vi "Box.vi"(4 "Position":cluster{"X":sgl, "Y":sgl, "Z":sgl}, 5 "Alpha":dbl=1.0, 7 "Color Box":u32(colorbox), 8 "error in (no error)":errorcluster, 9 "Size":T1, 10 "Name":string) -> (0 "error out":errorcluster, 3 "3D Object out":refnum<class "3D Object.lvclass">)   [LabVIEW 2015, in "3D Object.lvclass"]
uses:
  3D Object.lvclass
  <vilib>/picture/3D Picture Control/NI_3D Picture Control.lvlib
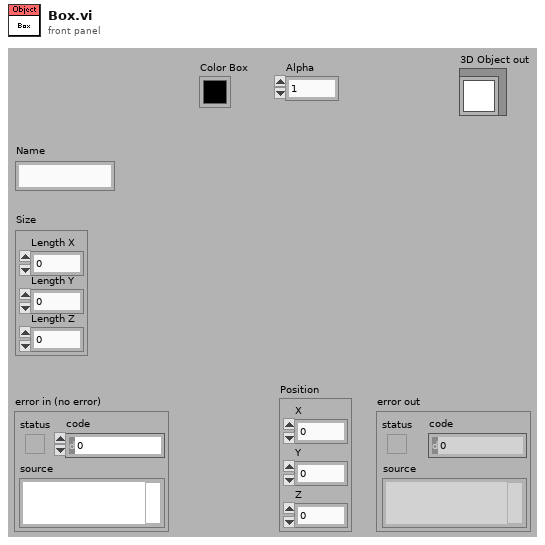
[diagram p1: front panel]
types:
  T1 = cluster{"Length X":sgl, "Length Y":sgl, "Length Z":sgl}
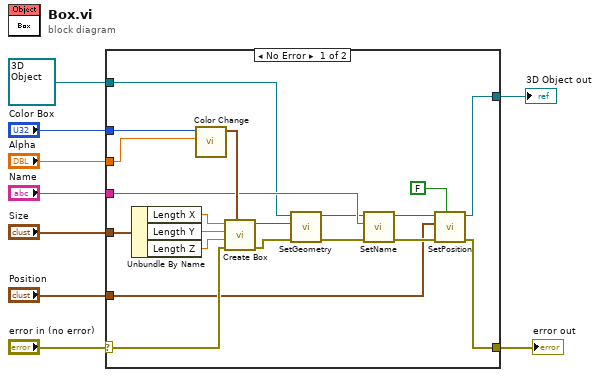
[diagram p0: block diagram]
diagram:
  n1 = case shown="No Error" "error in (no error)" {
    selector: "error in (no error)" -> [w13 w31]
    tunnel: [w24 w31] -> w8
    tunnel: refnum<class "3D Object.lvclass"> refnum ("3D Object in") -> [w12 w30]
    tunnel: [w23 w30] -> w6
    tunnel: "Color Box" -> [w26 _]
    tunnel: "Alpha" -> [w25 _]
    tunnel: "Position" -> [w11 _]
    tunnel: "Size" -> [w22 _]
    tunnel: "Name" -> [w18 _]
    frame No Error {
      n2 = Unbundle By Name(w22) -> ("Length X"=w21:sgl, "Length Y"=w20:sgl, "Length Z"=w19:sgl)
      n3 = call <vilib>:"Color Change.vi"("Alpha"=w25, "Color"=w26) -> ("RGBA"=w29:cluster{"R":sgl, "G":sgl, "B":sgl, "A":sgl})  [unwired: 9 out]
      n4 = call <vilib>:"Create Box.vi"("Color"=w29, "error in (no error)"=w13, "Length Z"=w19, "Length Y"=w20, "Length X"=w21) -> ("error out"=w27:errorcluster, "New Box Refnum"=w28:refnum<vi>)  [unwired: 5 out]
      n5 = call "SetGeometry.vi"("error in (no error)"=w27, "Geometry"=w28, "Object in"=w12) -> ("error out"=w16:errorcluster, "Object out"=w17:refnum<class "3D Object.lvclass">)  [unwired: 7 out]
      n6 = call "SetName.vi"("error in (no error)"=w16, "Name"=w18, "3D Object in"=w17) -> ("error out"=w14:errorcluster, "3D Object out"=w15:refnum<class "3D Object.lvclass">)  [unwired: 7 out]
      n7 = call "SetPosition.vi"("Relative?"=FALSE, "error in (no error)"=w14, "Position"=w11, "3D Object in"=w15) -> ("error out"=w24:errorcluster, "3D Object out"=w23:refnum<class "3D Object.lvclass">)  [unwired: 6 in]
    }
    frame Error {
    }
  }
  "error out" <- w8
  "3D Object out" <- w6
